vi "glb_LuaVIEW Configuration Globals.vi"() -> ()   [LabVIEW 2013]
doc: "LuaVIEW can be configured by setting these globals. This can be done from a bootstrap script (using the configure() function) or from LabVIEW."
panel:
  in  "task error logger":string
  in  "bootmode":string
  in  "task alternatives":refnum<vi>[](array[refnum])
  in  "mandatory import script":string
  in  "incite timeout":u32=2000
  in  "export timeout":u32=1000
  in  "custom info":string
  out "auto-init registry":bool=TRUE
  out "unload functions ASAP":bool
  in  "script search directories":path[](array[path])
  # "LuaVIEW can be configured by setting these globals. This can be done from a bootstrap script (using the configure() function) or from LabVIEW\non application startup (before starting scripts).\n\nThe default values are OK for running examples and other self-contained uses of Lua."
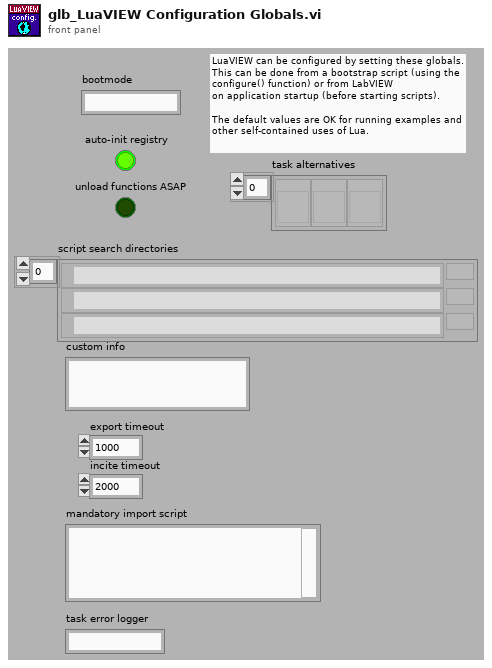
[diagram p1: front panel]
diagram:
